vi "Split Channel Name.vi"(11 "Channel Name":string) -> (1 "Split":bool, 2 "Child":string, 3 "Parent":string)   [LabVIEW 2021, in "CIFCoreCommon.lvlib"]
uses:
  CIFCoreCommon.lvlib
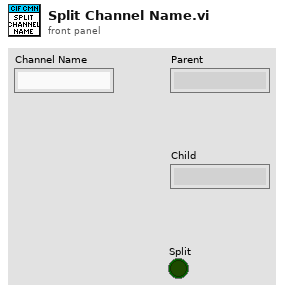
[diagram p1: front panel]
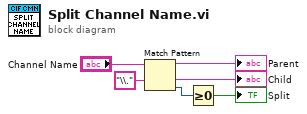
[diagram p0: block diagram]
diagram:
  n1 = Match Pattern(string="Channel Name", regular expression="\\.") -> (before substring=→"Parent":string, after substring=→"Child":string, offset past match=w2:i32)  [unwired: 1 in, 1 out]
  n2 = Greater Or Equal To 0?(x=w2) -> (x >= 0?=→"Split":bool)
